vi "APC_SIL0_HRL_Desktop.vi"() -> ()   [LabVIEW 2020]
uses:
  controls/APC_CombustionMetrics.ctl
  controls/APC_PcylDiag.ctl
  <vilib>/Utility/file.llb/Read Delimited Spreadsheet (DBL).vi
  <vilib>/Utility/file.llb/Write Delimited Spreadsheet (DBL).vi
panel:
  out "Pressure Trace":dbl[][](graph)
  out "size(s) 2":i32[](array[numeric])
  out "size(s)":i32[](array[numeric])
  out "all rows":dbl[][](array[numeric])
  out "IMEPg [bar]":dbl[](array[numeric])
  out "appended path":path
  in  "traces folder":path=path "C:/Users/RFSCtrlRoom/Desktop/Claude-Code-Projects/python-labview-controls-project/motored_set"
  out "PcylDiagWarningsAndErrors":T1[](array[typedef])
  out "Q":dbl[][](graph)
  out "HP filtered":dbl[][](graph)
  out "CombustionAnalysisCluster":T2={"IMEPn [bar]"=[6.211117999242393, 6.211117999242393, 6.211117999242393, 6.211117999242393, 6.211117999242393, 6.211117999242393], "IMEPg [bar]"=[6.4446479514403014, 6.4446479514403014, 6.4446479514403014, 6.4446479514403014, 6.4446479514403014, 6.4446479514403014], "MAPO [bar/CAD]"=[12.032314460918599, 12.032314460918599, 12.032314460918599, 12.032314460918599, 12.032314460918599, 12.032314460918599], "maxQ [J]"=[1738.4237704292323, 1738.4237704292323, 1738.4237704292323, 1738.4237704292323, 1738.4237704292323, 1738.4237704292323], "CA10  [CADATDC]"=[-3.3498503358307232, -3.3498503358307232, -3.3498503358307232, -3.3498503358307232, -3.3498503358307232, -3.3498503358307232], "CA50 [CADATDC]"=[5.494620967564458, 5.494620967564458, 5.494620967564458, 5.494620967564458, 5.494620967564458, 5.494620967564458], "CA90 [CADATDC]"=[nan, nan, nan, nan, nan, nan], "Pmax [bar]"=[65.51369273351828, 65.51369273351828, 65.51369273351828, 65.51369273351828, 65.51369273351828, 65.51369273351828], "IMEPstd [bar]"=[0.1430846822513861, 0.1430846822513861, 0.1430846822513861, 0.1430846822513861, 0.1430846822513861, 0.1430846822513861], "CA03  [CADATDC]"=[nan, nan, nan, nan, nan, nan], "CA97  [CADATDC]"=[nan, nan, nan, nan, nan, nan], "CA10CA90 [CADATDC]"=[nan, nan, nan, nan, nan, nan], "maxdpdCAD [bar/CAD]"=[nan, nan, nan, nan, nan, nan], "kappa_comp [-]"=[nan, nan, nan, nan, nan, nan], "kappa_exp [-]"=[nan, nan, nan, nan, nan, nan], "PMEP [bar]"=[nan, nan, nan, nan, nan, nan], "RI [-]"=[nan, nan, nan, nan, nan, nan]}
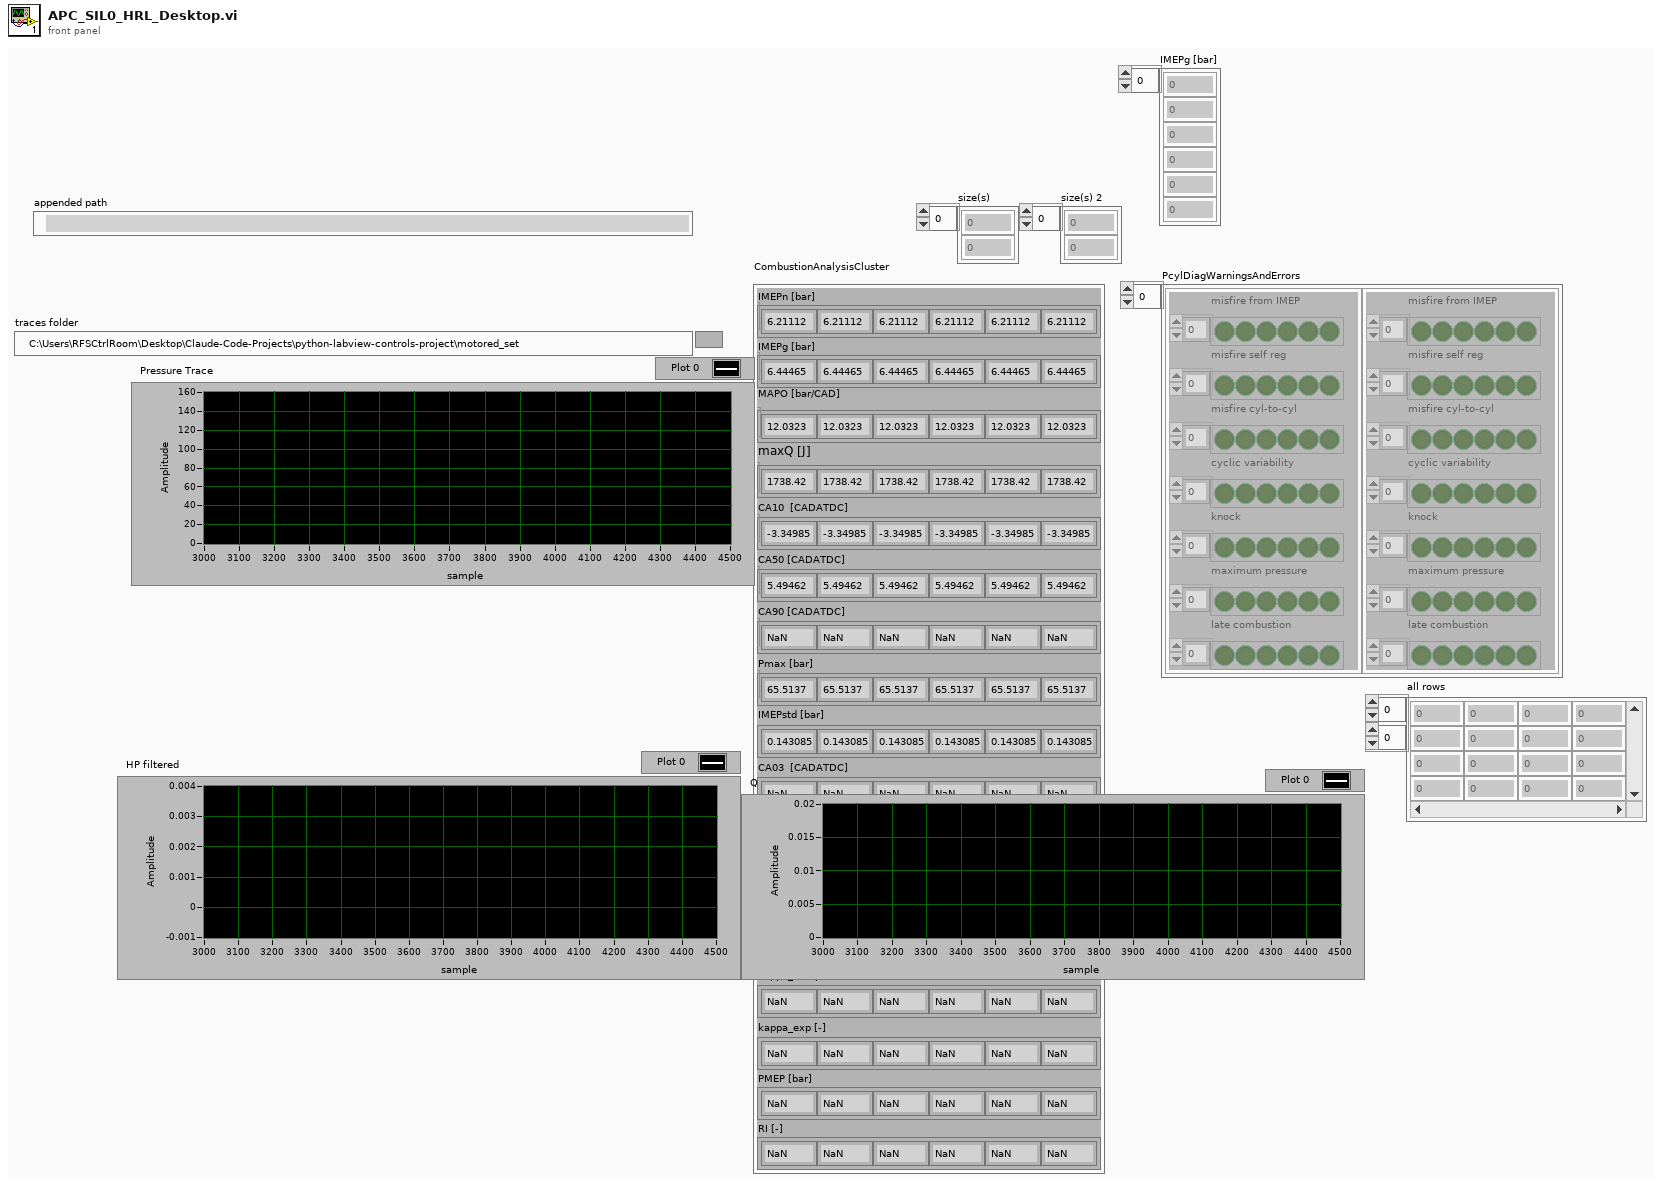
[diagram p1: front panel]
types:
  T1 = typedef "APC_PcylDiag.ctl" = cluster{"misfire from IMEP":bool[], "misfire self reg":bool[], "misfire cyl-to-cyl":bool[], "cyclic variability":bool[], "knock":bool[], "maximum pressure":bool[], "late combustion":bool[]}
  T2 = typedef "APC_CombustionMetrics.ctl" = cluster{"IMEPn [bar]":dbl[], "IMEPg [bar]":dbl[], "MAPO [bar/CAD]":dbl[], "maxQ [J]":dbl[], "CA10  [CADATDC]":dbl[], "CA50 [CADATDC]":dbl[], "CA90 [CADATDC]":dbl[], "Pmax [bar]":dbl[], "IMEPstd [bar]":dbl[], "CA03  [CADATDC]":dbl[], "CA97  [CADATDC]":dbl[], "CA10CA90 [CADATDC]":dbl[], "maxdpdCAD [bar/CAD]":dbl[], "kappa_comp [-]":dbl[], "kappa_exp [-]":dbl[], "PMEP [bar]":dbl[], "RI [-]":dbl[]}
  T3 = cluster{"IIR LowPass":cluster{"filter structure":enum32{"IIR 2nd Order", "IIR 4th Order"}, "Reverse Coefficients":dbl[], "Forward Coefficients":dbl[]}, "IIR HighPass":cluster{"filter structure":enum32{"IIR 2nd Order", "IIR 4th Order"}, "Reverse Coefficients":dbl[], "Forward Coefficients":dbl[]}}
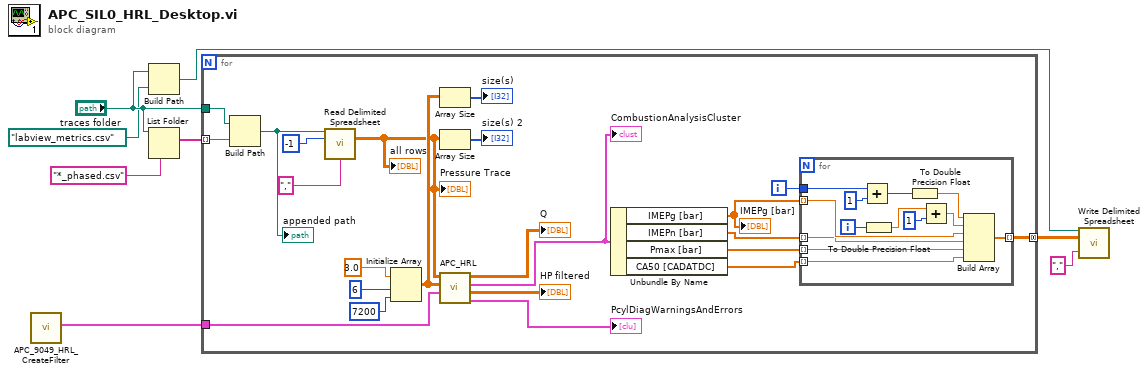
[diagram p0: block diagram]
diagram:
  n1 = call "APC_9049_HRL_CreateFilter.vi"() -> ("FilterCoefs"=w8:T3)  [unwired: 11 in]
  n2 = Build Path(base path="traces folder", name or relative path=path "labview_metrics.csv") -> (appended path=w1:path)
  n3 = List Folder(path="traces folder", pattern="*_phased.csv") -> (filenames=w6:string[])  [unwired: 2 in, 3 out]
  n4 = for {
    tunnel: w8 -> [w31]
    tunnel: w6 -> [w29] mode=indexing
    tunnel: "traces folder" -> [w30]
    tunnel: [w9] -> w5 mode=concatenating
    i -> [w10]
    n5 = Build Path(base path=w30, name or relative path=w29) -> (appended path=w28:path)
    "appended path" <- w28
    n6 = call-poly <vilib>:"Read Delimited Spreadsheet.vi"("file path (dialog if empty)"=w28, "number of rows (all:-1)"=-1, "delimiter (\\t)"="," ("delimiter (\\t)")) -> ("all rows"=w15:dbl[][])  [unwired: 7 in, 5 out]
    "all rows" <- w15
    "Pressure Trace" <- w15
    n7 = Initialize Array(3.0 ("element"), 6 ("dimension size"), 7200 ("dimension size")) -> (w20:dbl[][])
    n8 = Array Size(array=w20) -> (size(s)=→"size(s)":i32[])
    n9 = Array Size(array=w15) -> (size(s)=→"size(s) 2":i32[])
    n10 = call "APC_HRL.vi"("Pcyl"=w15, "exhaust pressure"=w20, "FilterCoefs"=w31) -> ("HRL [J]"=→"Q":dbl[][], "CombustionAnalysisCluster"=w24:T2, "HPfilt Pcyl"=→"HP filtered":dbl[][], "PcylDiagWarningsAndErrors"=→"PcylDiagWarningsAndErrors":T1[])  [unwired: 1 in, 1 out]
    "CombustionAnalysisCluster" <- w24
    n11 = Unbundle By Name(w24) -> ("IMEPg [bar]"=w14:dbl[], "IMEPn [bar]"=w13:dbl[], "Pmax [bar]"=w12:dbl[], "CA50 [CADATDC]"=w11:dbl[])
    "IMEPg [bar]" <- w14
    n12 = for {
      tunnel: w14 -> [w44] mode=indexing
      tunnel: w13 -> [w43] mode=indexing
      tunnel: w12 -> [w42] mode=indexing
      tunnel: w11 -> [w41] mode=indexing
      tunnel: w10 -> [w40]
      tunnel: [w36] -> w9 mode=indexing
      i -> [w38]
      n13 = Add(x=w40, y=1) -> (x+y=w37:i32)
      n14 = To Double Precision Float(number=w38) -> (double precision float=w33:dbl)
      n15 = To Double Precision Float(number=w37) -> (double precision float=w35:dbl)
      n16 = Add(x=w33, y=1) -> (x+y=w32:dbl)
      n17 = Build Array(w35, w32, w44, w43, w42, w41) -> (w36:dbl[])
    }
  }
  n18 = call-poly <vilib>:"Write Delimited Spreadsheet.vi"("file path (dialog if empty)"=w1, "2D data"=w5, "delimiter (\\t)"="," ("delimiter (\\t)")) -> ()  [unwired: 11 in, 2 out]
